vi "Manual Override Lock Control.vi"(0 "Buttons to Claim Manual Control Lock":refnum<vi>[](array[refnum]), 1 "Reactor Name":string, 5 "Indicators for Manual Control Lock Claimed":refnum<vi>[](array[refnum]), 7 "Current Locks":refnum<vi>, 9 "Lock Reentrance Rate":u32, 12 "Queue System":refnum<vi>, 13 "JSON Queue":refnum<vi>, 14 "Stop Program":refnum<vi>) -> ()   [LabVIEW 2022 SP3]
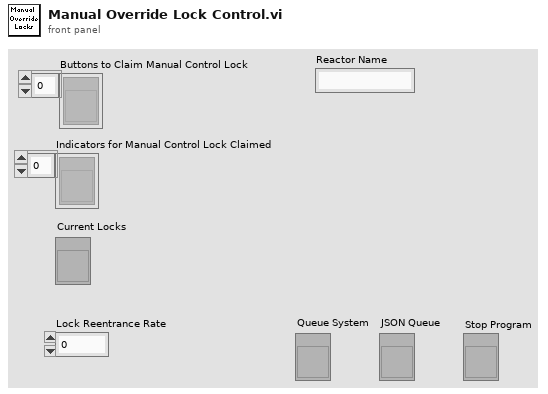
[diagram p1: front panel]
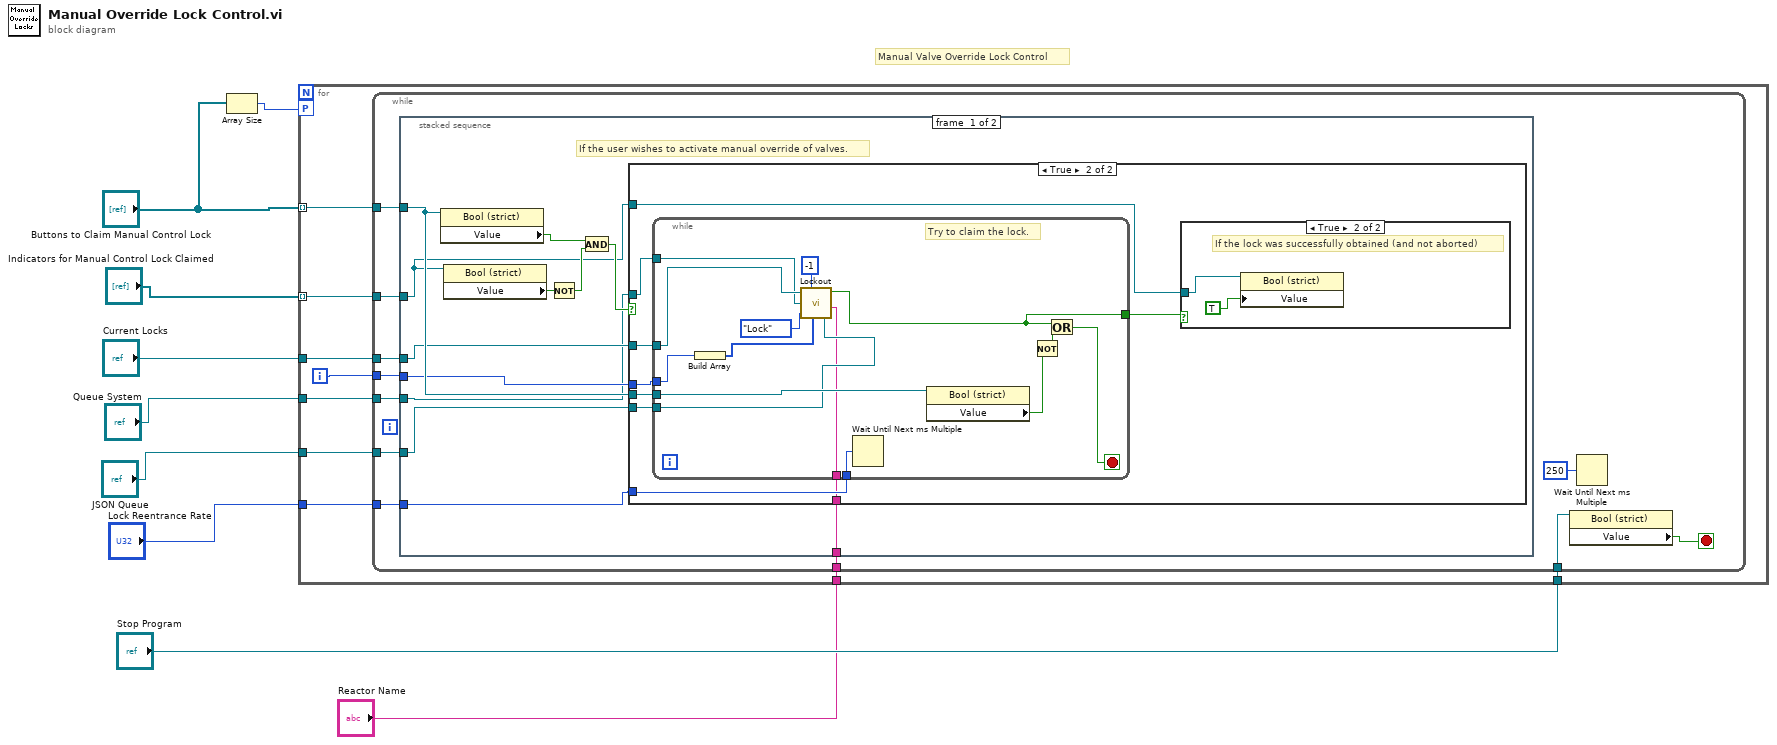
[diagram p0: block diagram]
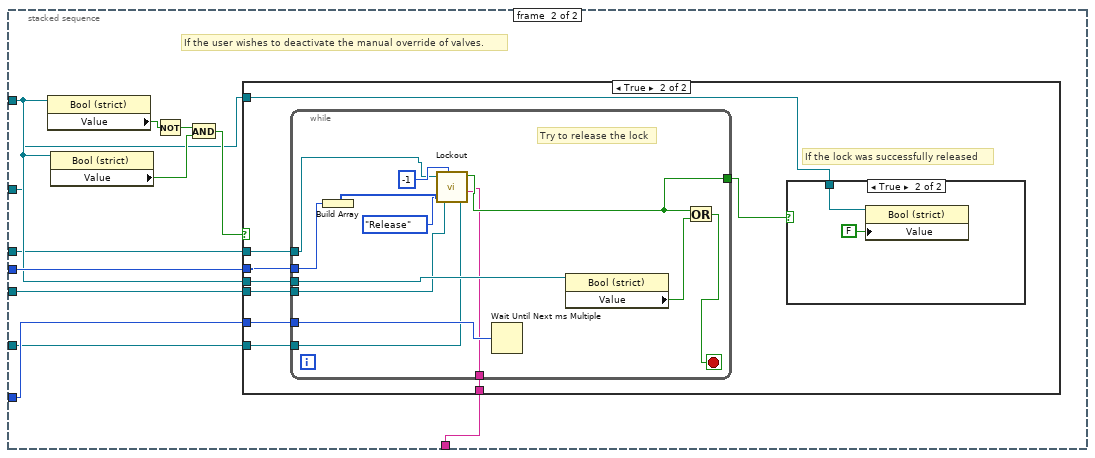
[diagram p4: hidden frame]
diagram:
  # "Manual Valve Override Lock Control"
  n1 = Array Size(array="Buttons to Claim Manual Control Lock") -> (size(s)=w2:i32)
  n2 = for {
    workers-P: w2 -> [_]
    tunnel: "Buttons to Claim Manual Control Lock" -> [w17] mode=indexing
    tunnel: "Indicators for Manual Control Lock Claimed" -> [w16] mode=indexing
    tunnel: "Stop Program" -> [w15]
    tunnel: "Lock Reentrance Rate" -> [w14]
    tunnel: "Current Locks" -> [w13]
    tunnel: "Queue System" -> [w12]
    tunnel: "JSON Queue" -> [w11]
    tunnel: "Reactor Name" -> [w10]
    i -> [w18]
    n3 = while {
      tunnel: w18 -> [w29]
      tunnel: w17 -> [w28]
      tunnel: w16 -> [w27]
      tunnel: w15 -> [w24]
      tunnel: w14 -> [w23]
      tunnel: w13 -> [w22]
      tunnel: w12 -> [w21]
      tunnel: w11 -> [w20]
      tunnel: w10 -> [w19]
      stop <- w25 stop-if-true
      n4 = stacked-sequence {
        tunnel: w29 -> [w35 w74]
        tunnel: w28 -> [w37 w73]
        tunnel: w27 -> [w36 w72]
        tunnel: w23 -> [w31 w71]
        tunnel: w22 -> [w34 w70]
        tunnel: w21 -> [w32 w69]
        tunnel: w20 -> [w33 w68]
        tunnel: w19 -> [w30 w67]
        frame #0 {
          # "If the user wishes to activate manual override of valves."
          n5 = property class="Bool (strict)"(reference=w37) -> ("Value"=w41:bool)  [unwired: 1 in, 2 out]
          n6 = property class="Bool (strict)"(reference=w36) -> ("Value"=w40:bool)  [unwired: 1 in, 2 out]
          n7 = Not(x=w40) -> (.not. x?=w39:bool)
          n8 = And(x=w41, y=w39) -> (x .and. y?=w38:bool)
          n9 = case shown="True" w38 {
            tunnel: w35 -> [_ w49]
            tunnel: w37 -> [_ w48]
            tunnel: w36 -> [_ w47]
            tunnel: w34 -> [_ w46]
            tunnel: w33 -> [_ w45]
            tunnel: w32 -> [_ w44]
            tunnel: w31 -> [_ w43]
            tunnel: w30 -> [_ w42]
            frame False {
              # "If not, do nothing."
            }
            frame True {
              n10 = while {
                tunnel: w49 -> [w53]
                tunnel: [w59] -> w50
                tunnel: w48 -> [w64]
                tunnel: w46 -> [w58]
                tunnel: w45 -> [w57]
                tunnel: w44 -> [w56]
                tunnel: w43 -> [w55]
                tunnel: w42 -> [w54]
                stop <- w65 stop-if-true
                # "Try to claim the lock."
                n11 = Build Array(w53) -> (w61:i32[])
                n12 = call "Lockout.vi"("Locks"=w58, "ID"=-1, "Queue System"=w56, "Request Type"=enum16{"Lock", "Release", "Check"}."Lock", "Request Array"=w61, "Reactor Name"=w54, "JSON Queue"=w57) -> ("Response"=w59:bool)  [unwired: 1 out]
                n13 = Wait Until Next ms Multiple(millisecond multiple=w55) -> ()  [unwired: 1 out]
                n14 = property class="Bool (strict)"(reference=w64) -> ("Value"=w66:bool)  [unwired: 1 in, 2 out]
                n15 = Not(x=w66) -> (.not. x?=w63:bool)
                n16 = Or(x=w59, y=w63) -> (x .or. y?=w65:bool)
              }
              n17 = case shown="True" w50 {
                tunnel: w47 -> [_ w51]
                frame False {
                }
                frame True {
                  # "If the lock was successfully obtained (and not aborted)"
                  n18 = property class="Bool (strict)"(reference=w51, "Value"=TRUE) -> ()  [unwired: 1 in, 2 out]
                }
              }
            }
          }
        }
        frame #1 {
          # "If the user wishes to deactivate the manual override of valves."
          n19 = property class="Bool (strict)"(reference=w73) -> ("Value"=w78:bool)  [unwired: 1 in, 2 out]
          n20 = property class="Bool (strict)"(reference=w72) -> ("Value"=w77:bool)  [unwired: 1 in, 2 out]
          n21 = Not(x=w78) -> (.not. x?=w76:bool)
          n22 = And(x=w76, y=w77) -> (x .and. y?=w75:bool)
          n23 = case shown="True" w75 {
            tunnel: w74 -> [_ w84]
            tunnel: w73 -> [_ w87]
            tunnel: w72 -> [_ w86]
            tunnel: w71 -> [_ w83]
            tunnel: w70 -> [_ w82]
            tunnel: w69 -> [_ w81]
            tunnel: w68 -> [_ w80]
            tunnel: w67 -> [_ w79]
            frame False {
            }
            frame True {
              # "If the lock was successfully released"
              n24 = while {
                tunnel: w84 -> [w101]
                tunnel: w87 -> [w100]
                tunnel: [w95] -> w85
                tunnel: w83 -> [w94]
                tunnel: w82 -> [w93]
                tunnel: w81 -> [w92]
                tunnel: w80 -> [w91]
                tunnel: w79 -> [w90]
                stop <- w99 stop-if-true
                # "Try to release the lock"
                n25 = Build Array(w101) -> (w97:i32[])
                n26 = call "Lockout.vi"("Locks"=w93, "ID"=-1, "Queue System"=w92, "Request Type"=enum16{"Lock", "Release", "Check"}."Release", "Request Array"=w97, "Reactor Name"=w90, "JSON Queue"=w91) -> ("Response"=w95:bool)  [unwired: 1 out]
                n27 = Wait Until Next ms Multiple(millisecond multiple=w94) -> ()  [unwired: 1 out]
                n28 = property class="Bool (strict)"(reference=w100) -> ("Value"=w102:bool)  [unwired: 1 in, 2 out]
                n29 = Or(x=w95, y=w102) -> (x .or. y?=w99:bool)
              }
              n30 = case shown="True" w85 {
                tunnel: w86 -> [_ w88]
                frame False {
                }
                frame True {
                  n31 = property class="Bool (strict)"(reference=w88, "Value"=FALSE) -> ()  [unwired: 1 in, 2 out]
                }
              }
            }
          }
        }
      }
      n32 = property class="Bool (strict)"(reference=w24) -> ("Value"=w25:bool)  [unwired: 1 in, 2 out]
      n33 = Wait Until Next ms Multiple(millisecond multiple=u32 250) -> ()  [unwired: 1 out]
    }
  }
